vi "array.vi"() -> ()   [LabVIEW 2020]
uses:
  02663f7c-4c89-4829-99cc-8eb967d08cdc.vi
  <vilib>/Comparison/Equal/Equal Functor/Equal Functor.lvclass
panel:
  out "x+y":dbl[](array[numeric])
  in  "Array 5":dbl[](array[numeric])
  in  "Array 4":dbl[](array[numeric])
  out "inc":dbl[](array[numeric])
  in  "n 2":i32
  out "array (last n elements first) 2":dbl[](array[numeric])
  out "array (last n elements first)":dbl[](array[numeric])
  in  "n":i32
  out "second subarray":dbl[](array[numeric])
  out "first subarray":dbl[](array[numeric])
  in  "index 4":i32
  in  "start index (0)":i32
  out "index of element":i32
  in  "element 6":dbl
  out "reversed array":dbl[](array[numeric])
  out "output array":dbl[](array[numeric])
  in  "dimension size 2":i32
  out "max index(es)":i32
  out "min index(es)":i32
  out "min value":dbl
  out "max value":dbl
  out "subarray":dbl[](array[numeric])
  in  "index 3":i32
  in  "length 2":i32
  out "deleted portion":dbl[](array[numeric])
  out "array w/ subset deleted":dbl[](array[numeric])
  in  "index 2":i32
  in  "length":i32
  out "element 5":dbl
  in  "index":i32
  out "size(s)":i32
  out "appended array":dbl[](array[numeric])
  in  "element 4":dbl
  in  "element 3":dbl
  in  "element 2":dbl
  out "initialized array":dbl[](array[numeric])
  in  "dimension size":i32
  in  "element":dbl
  in  "Array 3":string[](array[string])
  in  "Array 2":bool[](array[boolean])
  in  "Array":dbl[](array[numeric])
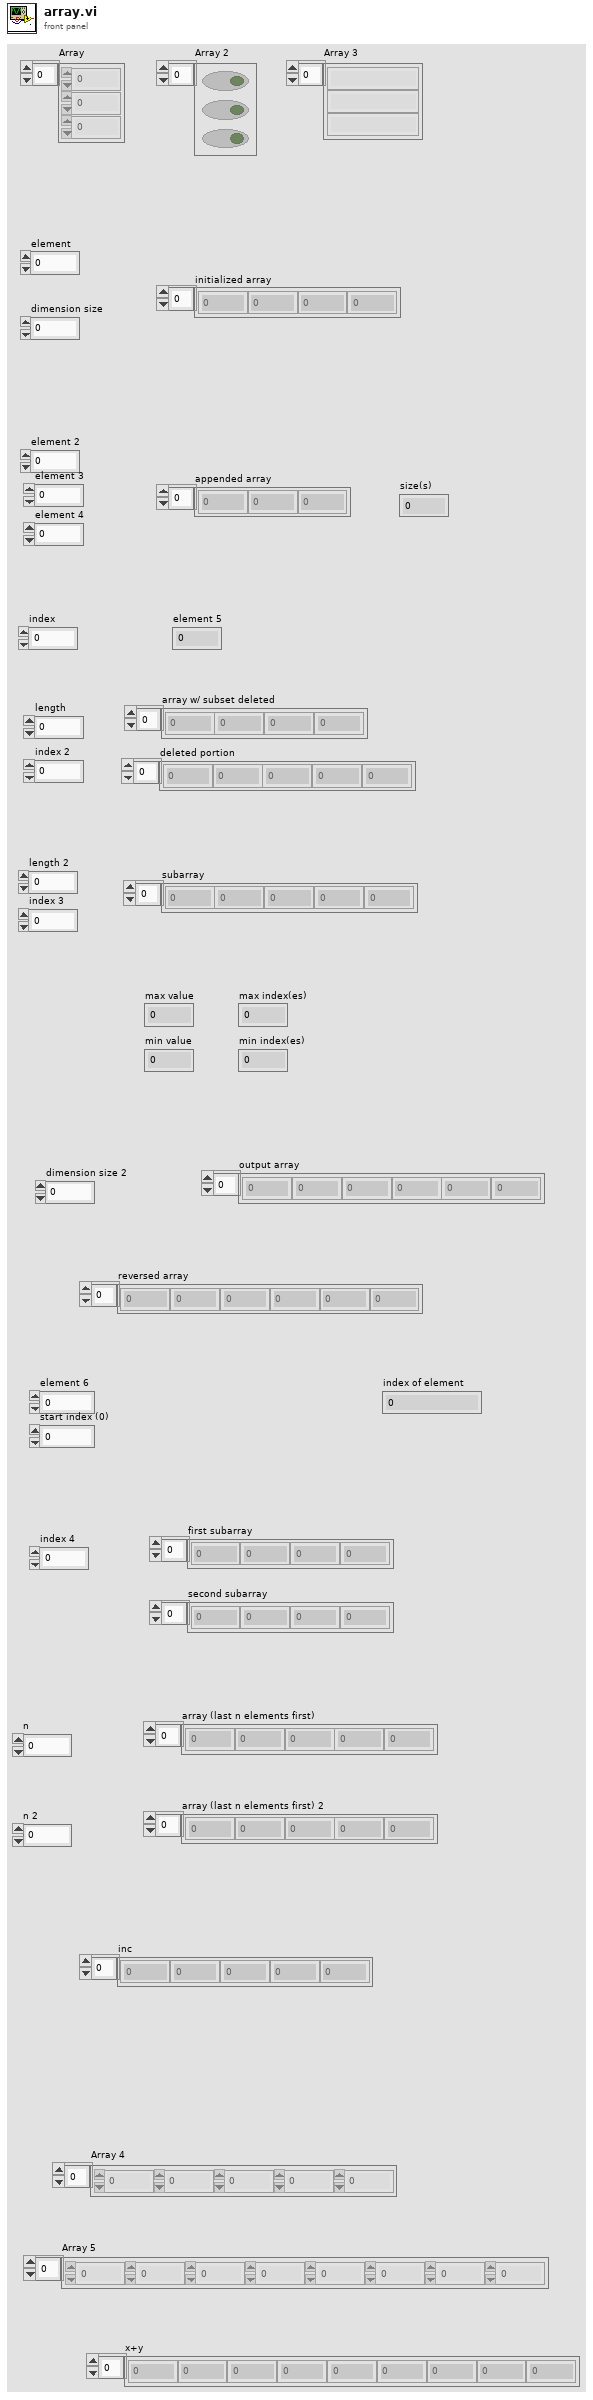
[diagram p1: front panel]
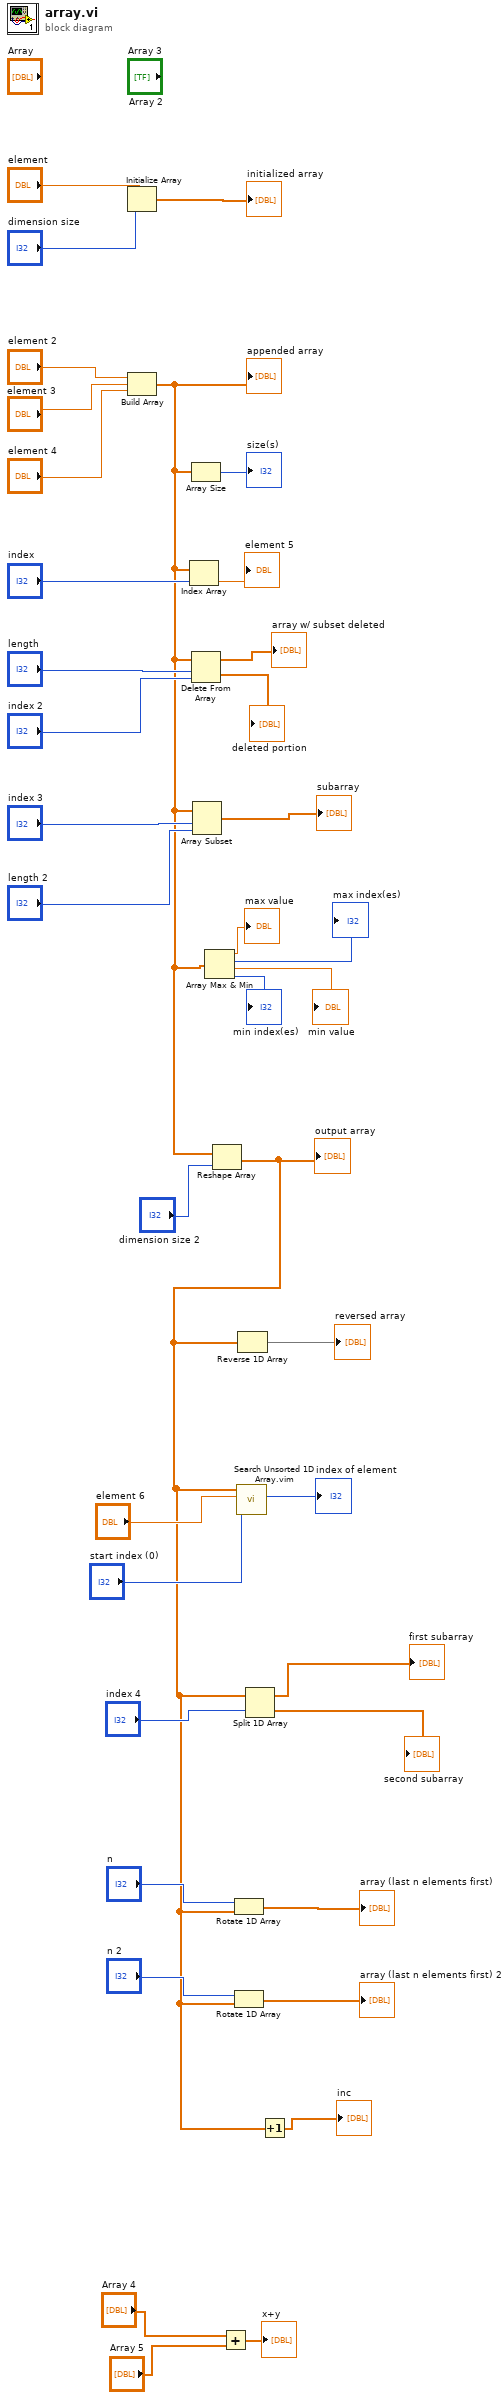
[diagram p0: block diagram]
diagram:
  n1 = Initialize Array("element", "dimension size") -> (→"initialized array":dbl[])
  n2 = Build Array("element 2", "element 3", "element 4") -> (w17:dbl[])
  "appended array" <- w17
  n3 = Index Array(array=w17, index="index") -> (element=→"element 5":dbl)
  n4 = Array Size(array=w17) -> (size(s)=→"size(s)":i32)
  n5 = Delete From Array(array=w17, length="length", index="index 2") -> (deleted portion=→"deleted portion":dbl[], array with subset deleted=→"array w/ subset deleted":dbl[])
  n6 = Array Subset(array=w17, index="index 3", length="length 2") -> (→"subarray":dbl[])
  n7 = Array Max & Min(array=w17) -> (max value=→"max value":dbl, max index (indices)=→"max index(es)":i32, min value=→"min value":dbl, min index (indices)=→"min index(es)":i32)
  n8 = Reshape Array(w17, "dimension size 2") -> (w5:dbl[])
  "output array" <- w5
  n9 = Add(x="Array 4", y="Array 5") -> (x+y=→"x+y":dbl[])
  n10 = Rotate 1D Array(1:w5, 2:"n") -> (0:→"array (last n elements first)":dbl[])
  n11 = Rotate 1D Array(1:w5, 2:"n 2") -> (0:→"array (last n elements first) 2":dbl[])
  n12 = call "Search Unsorted 1D Array.vim"("start index (0)"="start index (0)", "element"="element 6", "unsorted 1D array"=w5) -> ("index of element"=→"index of element":i32)  [unwired: 8 in]
  n13 = Reverse 1D Array(array=w5) -> (reversed array=→"reversed array":dbl[])
  n14 = Split 1D Array(array=w5, index="index 4") -> (first subarray=→"first subarray":dbl[], second subarray=→"second subarray":dbl[])
  n15 = Increment(x=w5) -> (x+1=→"inc":dbl[])
